vi "Initialise the Error log Based on Cycle number.vi"(8 "error in (no error)":errorcluster, 11 "Error Log in":refnum<class "Error Log.lvclass">) -> (0 "error out":errorcluster, 3 "Error Log out":refnum<class "Error Log.lvclass">)   [LabVIEW 2023, in "Data Analysis.lvlib" / "Error Log.lvlib" / "Error Log.lvclass"]
uses:
  Error Log.lvclass
  Error Log.lvclass/Error Log.ctl
  HardwareAbstractionLayer_LVOOP/Database/Database.lvclass
  Data Analysis.lvlib
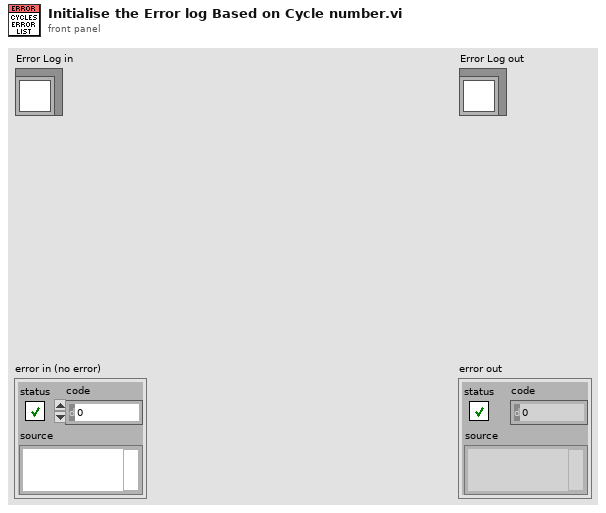
[diagram p1: front panel]
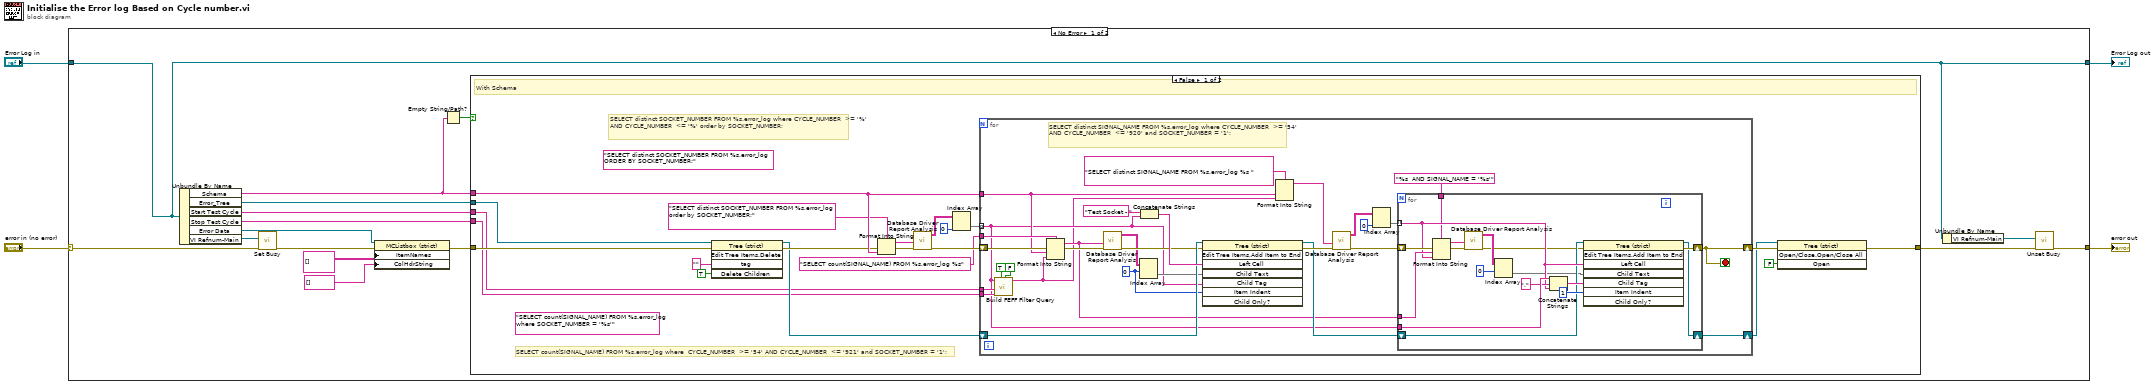
[diagram p0: block diagram]
diagram:
  n1 = case shown="No Error" "error in (no error)" {
    selector: "error in (no error)" -> [w10 w90]
    tunnel: [w7 w90] -> w3
    tunnel: [w5 w89] -> w1
    tunnel: "Error Log in" -> [w5 w89]
    frame No Error {
      n2 = Unbundle By Name(w5) -> ("Schema"=w15:string, "Error_Tree"=w20:refnum<vi>, "Start Test Cycle"=w13:string, "Stop Test Cycle"=w12:string, "Error Data"=w19:refnum<vi>, "VI Refnum-Main"=w11:refnum<vi>)
      n3 = call <vilib>:"Set Busy.vi"("error in (no error)"=w10, "VI reference (current VI)"=w11) -> ("error out"=w9:errorcluster)  [unwired: 8 in, 1 out]
      n4 = property class="MCListbox (strict)"(reference=w19, error in=w9, "ItemNames"=string[][] [] ("Item Names"), "ColHdrString"=string[] [] ("Column Header Strings[]")) -> (error out=w16:errorcluster)  [unwired: 1 out]
      n5 = Empty String/Path?(string/path=w15) -> (empty?=w14:bool)
      n6 = case shown="False" w14 {
        tunnel: [w41 w88] -> w8
        tunnel: w20 -> [w40 _]
        tunnel: w16 -> [w38 w88]
        tunnel: w15 -> [w39 _]
        tunnel: w13 -> [w22 _]
        tunnel: w12 -> [w21 _]
        frame False {
          (unwired) "SELECT count(SIGNAL_NAME) FROM %s.error_log where SOCKET_NUMBER = '%s'" ("SQL query")
          (unwired) "SELECT distinct SOCKET_NUMBER FROM %s.error_log ORDER BY SOCKET_NUMBER;" ("SQL query")
          # "SELECT count(SIGNAL_NAME) FROM %s.error_log where  CYCLE_NUMBER  >= '54' AND CYCLE_NUMBER  <= '921' and SOCKET_NUMBER = '1';"
          # "SELECT distinct SOCKET_NUMBER FROM %s.error_log where CYCLE_NUMBER  >= '%' AND CYCLE_NUMBER  <= '%' order by SOCKET_NUMBER;"
          # "With Schema"
          n7 = invoke on="Invoke Node" class="Tree (strict)" method="Edit Tree Items.Delete"(reference=w40, error in=w38, "tag"="" ("Tag"), "Delete Children"=TRUE ("Delete Children?")) -> (reference out=w23:refnum<vi>, error out=w35:errorcluster)  [unwired: 1 in, 3 out]
          n8 = Format Into String(format string="SELECT distinct SOCKET_NUMBER FROM %s.error_log  order by SOCKET_NUMBER;" ("SQL query"), error in=w35, w39) -> (resulting string=w32:string, error out=w36:errorcluster)  [unwired: 1 in]
          n9 = call "Database Driver Report Analysis.vi"("error in"=w36, "SQL query"=w32) -> ("error out"=w28:errorcluster, "data"=w29:string[][])  [unwired: 6 in, 2 out]
          n10 = Index Array(array=w29, index (col)=0 ("disabled index (col)")) -> (element=w30:string[])  [unwired: 1 in]
          n11 = for {
            tunnel: w30 -> [w45] mode=indexing
            shift-right: [w68] -> w37
            shift-left: w28 -> [w56]
            tunnel: w39 -> [w53]
            shift-right: [w58] -> w25
            shift-left: w23 -> [w60]
            tunnel: "SELECT count(SIGNAL_NAME) FROM %s.error_log %s" ("SQL query") -> [w54]
            tunnel: w22 -> [w47]
            tunnel: w21 -> [w46]
            stop <- w68 stop-if-true
            w50 = 0 ("index (row)")
            # "SELECT distinct SIGNAL_NAME FROM %s.error_log where CYCLE_NUMBER  >= '54' AND CYCLE_NUMBER  <= '920' and SOCKET_NUMBER = '1';"
            n12 = call "Build FEFF Filter Query.vi"("ORDER BY needed?(Yes)"=FALSE, "WHERE needed?(Yes)"=TRUE, "Stop Test Cycle"=w46, "Start Test Cycle"=w47, "Test Socket"=w45) -> ("String"=w43:string)  [unwired: 6 in]
            n13 = Format Into String(format string=w54, error in=w56, w53, w43) -> (resulting string=w49:string, error out=w55:errorcluster)  [unwired: 1 in]
            n14 = call "Database Driver Report Analysis.vi"("error in"=w55, "SQL query"=w49) -> ("error out"=w57:errorcluster, "data"=w52:string[][])  [unwired: 6 in, 2 out]
            n15 = Index Array(array=w52, index (row)=w50) -> (element=w51:string[])  [unwired: 1 in]
            n16 = Concatenate Strings("Test Socket - " ("element"), w45) -> (w69:string)
            n17 = invoke on="Invoke Node" class="Tree (strict)" method="Edit Tree Items.Add Item to End"(reference=w60, error in=w57, "Left Cell"=w69, "Child Text"=w51, "Child Tag"=w45, "Item Indent"=w50) -> (reference out=w59:refnum<vi>, error out=w67:errorcluster)  [unwired: 2 in, 6 out]
            n18 = Format Into String(format string="SELECT distinct SIGNAL_NAME FROM %s.error_log %s " ("SQL query"), w53, w43) -> (resulting string=w64:string)  [unwired: 2 in, 1 out]
            n19 = call "Database Driver Report Analysis.vi"("error in"=w67, "SQL query"=w64) -> ("error out"=w66:errorcluster, "data"=w62:string[][])  [unwired: 6 in, 2 out]
            n20 = Index Array(array=w62, index (col)=0 ("disabled index (col)")) -> (element=w61:string[])  [unwired: 1 in]
            n21 = for {
              shift-right: [w87] -> w68
              shift-left: w66 -> [w81]
              tunnel: w61 -> [w79] mode=indexing
              tunnel: w45 -> [w85]
              shift-right: [w82] -> w58
              shift-left: w59 -> [w77]
              tunnel: w49 -> [w80]
              tunnel: "%s  AND SIGNAL_NAME = '%s'" ("format string") -> [w78]
              n22 = Format Into String(format string=w78, error in=w81, w80, w79) -> (resulting string=w71:string, error out=w74:errorcluster)  [unwired: 1 in]
              n23 = call "Database Driver Report Analysis.vi"("error in"=w74, "SQL query"=w71) -> ("error out"=w73:errorcluster, "data"=w76:string[][])  [unwired: 6 in, 2 out]
              n24 = Index Array(array=w76, index (row)=0) -> (element=w72:string[])  [unwired: 1 in]
              n25 = Concatenate Strings(w85, "." ("string"), w79) -> (w83:string)
              n26 = invoke on="Invoke Node" class="Tree (strict)" method="Edit Tree Items.Add Item to End"(reference=w77, error in=w73, "Left Cell"=w79, "Child Text"=w72, "Child Tag"=w83, "Item Indent"=1 ("New Item Indentation")) -> (reference out=w82:refnum<vi>, error out=w87:errorcluster)  [unwired: 2 in, 6 out]
            }
          }
          n27 = invoke on="Invoke Node" class="Tree (strict)" method="Open/Close.Open/Close All"(reference=w25, error in=w37, "Open"=FALSE ("Open?")) -> (error out=w41:errorcluster)  [unwired: 1 in, 3 out]
        }
        frame True, Default {
        }
      }
      n28 = Unbundle By Name(w5) -> ("VI Refnum-Main"=w6:refnum<vi>)
      n29 = call <vilib>:"Unset Busy.vi"("error in (no error)"=w8, "VI reference (current VI)"=w6) -> ("error out"=w7:errorcluster)  [unwired: 9 in]
    }
    frame Error {
    }
  }
  "error out" <- w3
  "Error Log out" <- w1
